vi "Read All Data.vi"(8 "Error In":errorcluster, 11 "Leap Handle":T14) -> (0 "Error Out":errorcluster, 1 "Leap Connected?":bool, 2 "Frame":T1, 3 "Leap Handle":T14)   [LabVIEW 2011, in "LMH-Leap.lvlib"]
doc: "<b>Leap Read</b> requests and parses a <b>Frame</b> of data from the Leap Motion Controller. All the data associated with the Frame is organized into a LabVIEW cluster for accessibility.\n\nSpecifics about the data in the Frame cluster can be found by going to <b>Help » Leap Motion Controller Help</b> inside of LabVIEW"
uses:
  LMH-Leap.lvlib
  Private/Type Defs/Leap Handle.ctl
  C:/github/makerhub/Leap/LabVIEW/vi.lib/MakerHub/Leap/Private/Libs/LeapCSharp.NET3.5.dll
  Private/Libs/LeapCSharp.NET3.5.dll
  Private/Type Defs/Frame.ctl
  Private/Type Defs/Gesture Key Tap.ctl
  Private/Type Defs/Gesture Common.ctl
  Private/Type Defs/Gesture Type.ctl
  Private/Type Defs/Gesture State.ctl
  Private/Type Defs/Vector.ctl
  Private/Type Defs/Gesture Circle.ctl
  Private/Type Defs/Gesture Screen Tap.ctl
  Private/Type Defs/Gesture Swipe.ctl
  Private/Type Defs/Hand.ctl
  Private/Type Defs/Pointable.ctl
  Private/Type Defs/Pointable Type.ctl
  Private/Type Defs/Pointable Zone.ctl
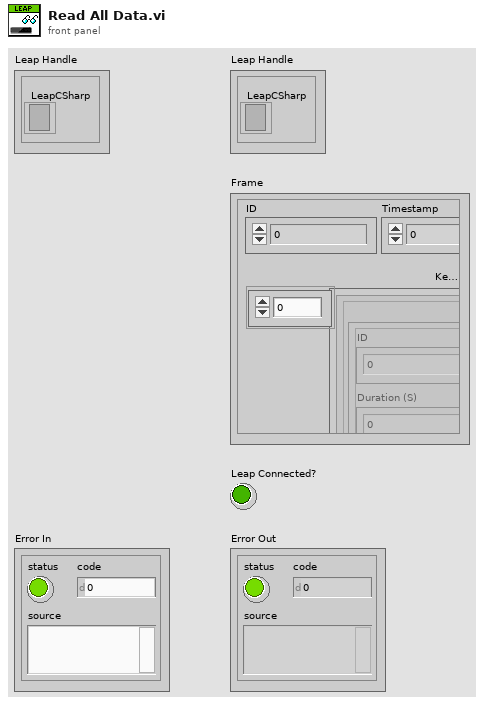
[diagram p1: front panel]
types:
  T1 = typedef "LMH-Leap.lvlib/Frame.ctl" = cluster{"ID":i64, "Timestamp":i64, "Current FPS":dbl, "Key Tap Gestures":T2[], "Circle Gestures":T7[], "Screen Tap Gestures":T8[], "Swipe Gestures":T9[], "Hands":T10[]}
  T2 = typedef "LMH-Leap.lvlib/Gesture Key Tap.ctl" = cluster{"Common":T3, "Direction":T6, "Position":T6, "Progress":dbl}
  T3 = typedef "LMH-Leap.lvlib/Gesture Common.ctl" = cluster{"ID":dbl, "Duration (S)":dbl, "Gesture Type":T4, "Gesture State":T5}
  T4 = typedef "LMH-Leap.lvlib/Gesture Type.ctl" = enum16{"Invalid", "Swipe", "Circle", "Screen Tap", "Key Tap"}
  T5 = typedef "LMH-Leap.lvlib/Gesture State.ctl" = enum16{"Invalid", "Start", "Update", "Stop"}
  T6 = typedef "LMH-Leap.lvlib/Vector.ctl" = cluster{"Pitch":sgl, "Yaw":sgl, "Roll":sgl, "Magnitude":sgl, "XYZ":sgl[]}
  T7 = typedef "LMH-Leap.lvlib/Gesture Circle.ctl" = cluster{"Common":T3, "Center":T6, "Normal":T6, "Progress":dbl, "Radius":dbl}
  T8 = typedef "LMH-Leap.lvlib/Gesture Screen Tap.ctl" = cluster{"Common":T3, "Direction":T6, "Position":T6, "Progress":dbl}
  T9 = typedef "LMH-Leap.lvlib/Gesture Swipe.ctl" = cluster{"Common":T3, "Direction":T6, "Position":T6, "Start Position":T6, "Speed":dbl}
  T10 = typedef "LMH-Leap.lvlib/Hand.ctl" = cluster{"Palm Normal":T6, "Palm Position":T6, "Palm Velocity":T6, "Direction":T6, "Palm Position (Stabilized)":T6, "Sphere Center":T6, "Pointables":T11[], "ID":i32, "Time Visible":sgl, "Sphere Radius":sgl}
  T11 = typedef "LMH-Leap.lvlib/Pointable.ctl" = cluster{"Type":T12, "Touch Zone":T13, "ID":i32, "Length":dbl, "Width":dbl, "Time Visible":dbl, "Touch Distance":dbl, "Direction":T6, "Tip Position":T6, "Tip Velocity":T6, "Tip Position (Stabilized)":T6}
  T12 = typedef "LMH-Leap.lvlib/Pointable Type.ctl" = enum16{"Finger", "Tool"}
  T13 = typedef "LMH-Leap.lvlib/Pointable Zone.ctl" = enum16{"None", "Hovering", "Touching"}
  T14 = typedef "LMH-Leap.lvlib/Leap Handle.ctl" = cluster{"LeapCSharp":refnum<k24>}
  T15 = typedef "LMH-Leap.lvlib/All Gestures.ctl" = cluster{"Swipe Gestures":T9[], "Circle Gestures":T7[], "Screen Tap Gestures":T8[], "Key Tap Gestures":T2[]}
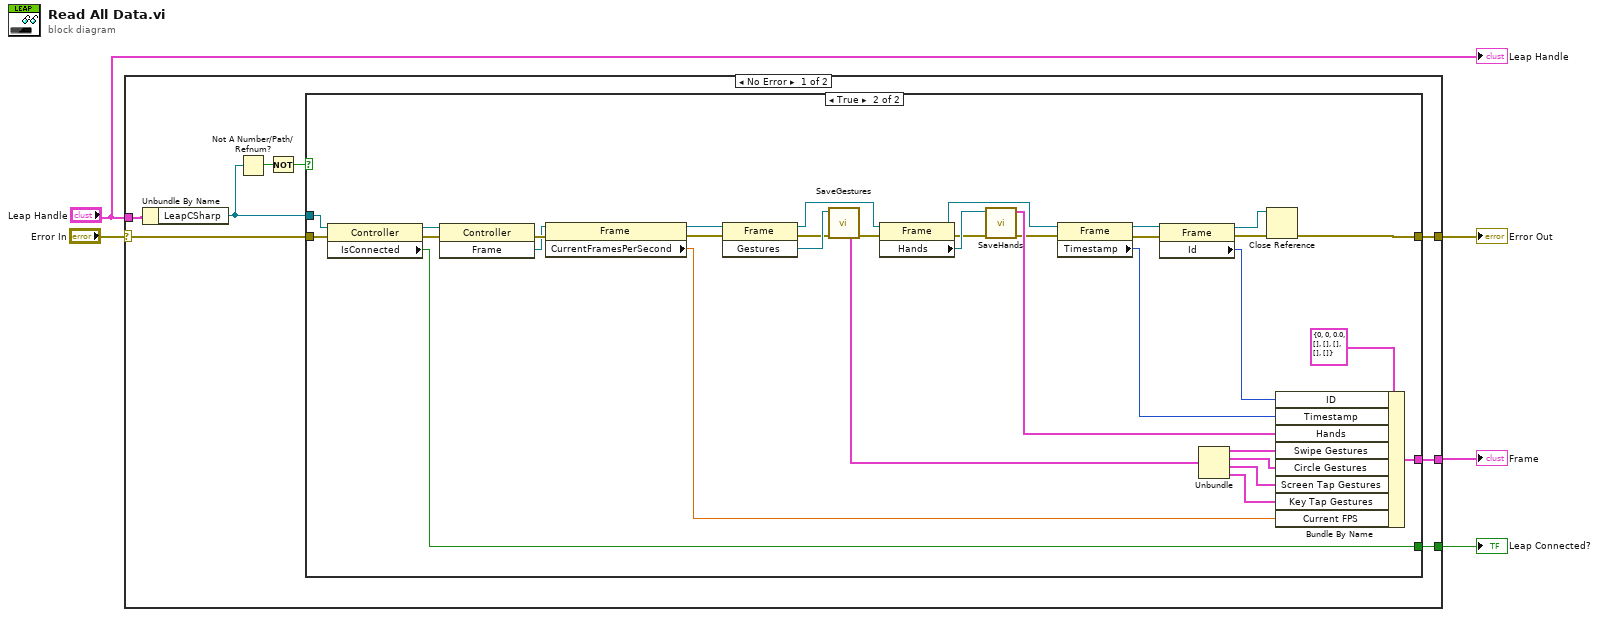
[diagram p0: block diagram]
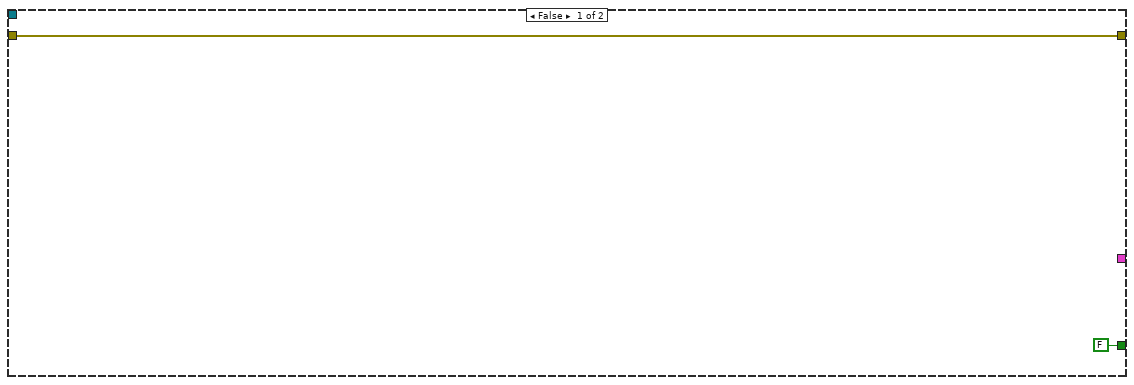
[diagram p2: hidden frame]
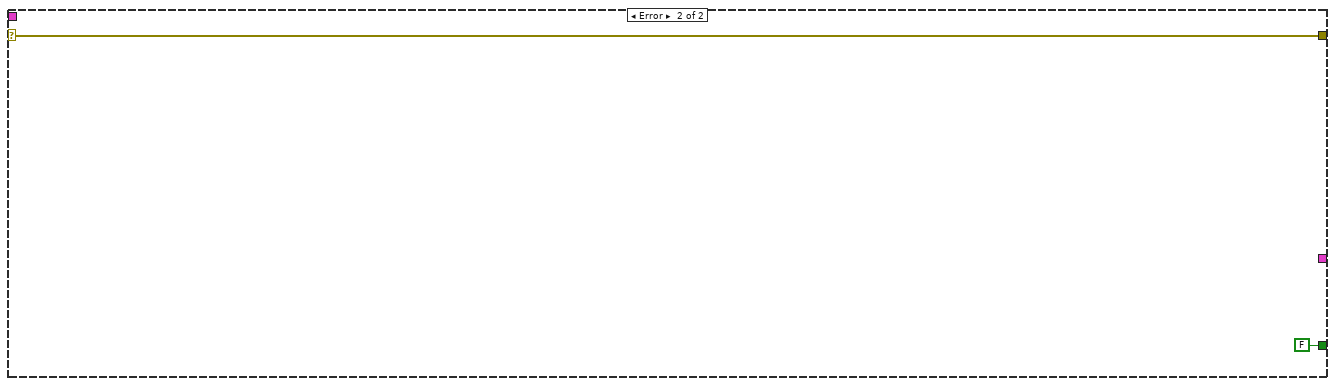
[diagram p3: hidden frame]
diagram:
  n1 = case shown="No Error" "Error In" {
    selector: "Error In" -> [w11 w50]
    tunnel: "Leap Handle" -> [w13 _]
    tunnel: [w12 _] -> w4
    tunnel: [w10 w50] -> w2
    tunnel: [w6 FALSE ("IsConnected")] -> w1
    frame No Error {
      n2 = Unbundle By Name(w13) -> ("LeapCSharp"=w7:refnum<k24>)
      n3 = Not A Number/Path/Refnum?(number/path/refnum=w7) -> (NaN/Path/Refnum?=w9:bool)
      n4 = Not(x=w9) -> (.not. x?=w8:bool)
      n5 = case shown="True" w8 {
        tunnel: [_ w48] -> w12
        tunnel: w7 -> [_ w33]
        tunnel: w11 -> [w15 w30]
        tunnel: [w15 w45] -> w10
        tunnel: [FALSE ("IsConnected") w34] -> w6
        frame False {
        }
        frame True {
          n6 = property class="Controller"(reference=w33, error in=w30) -> (reference out=w32:refnum<k24>, error out=w31:errorcluster, "IsConnected"=w34:bool)
          n7 = invoke class="Controller" method="Frame"(reference=w32, error in=w31) -> (error out=w27:errorcluster, "Frame"=w26:refnum<k24>)  [unwired: 1 in, 1 out]
          n8 = property class="Frame"(reference=w26, error in=w27) -> (reference out=w24:refnum<k24>, error out=w25:errorcluster, "CurrentFramesPerSecond"=w35:sgl)
          n9 = invoke class="Frame" method="Gestures"(reference=w24, error in=w25) -> (reference out=w22:refnum<k24>, error out=w28:errorcluster, "Gestures"=w44:refnum<k24>)  [unwired: 1 in]
          n10 = call "SaveGestures.vi"("Error In"=w28, ".NET Refnum in"=w44) -> ("Error Out"=w23:errorcluster, "All Gestures"=w43:T15)  [unwired: 8 in]
          n11 = property class="Frame"(reference=w22, error in=w23) -> (reference out=w21:refnum<k24>, error out=w29:errorcluster, "Hands"=w47:refnum<k24>)
          n12 = call "SaveHands.vi"("Error In"=w29, ".NET Refnum in"=w47) -> ("Error Out"=w20:errorcluster, "Hands"=w38:T10[])  [unwired: 8 in]
          n13 = property class="Frame"(reference=w21, error in=w20) -> (reference out=w19:refnum<k24>, error out=w18:errorcluster, "Timestamp"=w37:i64)
          n14 = property class="Frame"(reference=w19, error in=w18) -> (reference out=w17:refnum<k24>, error out=w16:errorcluster, "Id"=w36:i64)
          n15 = Unbundle(w43) -> ("Swipe Gestures"=w42:T9[], "Circle Gestures"=w41:T7[], "Screen Tap Gestures"=w40:T8[], "Key Tap Gestures"=w39:T2[])
          n16 = Close Reference(reference=w17, error in (no error)=w16) -> (error out=w45:errorcluster)
          n17 = Bundle By Name(cluster=T1 {"ID"=0, "Timestamp"=0, "Current FPS"=0.0, "Key Tap Gestures"=[], "Circle Gestures"=[], "Screen Tap Gestures"=[], "Swipe Gestures"=[], "Hands"=[]} ("Frame"), "ID"=w36, "Timestamp"=w37, "Hands"=w38, "Swipe Gestures"=w42, "Circle Gestures"=w41, "Screen Tap Gestures"=w40, "Key Tap Gestures"=w39, "Current FPS"=w35) -> (w48:T1)
        }
      }
    }
    frame Error {
    }
  }
  "Frame" <- w4
  "Error Out" <- w2
  "Leap Connected?" <- w1
  "Leap Handle" <- "Leap Handle"
